vi "sendToAll.vi"(8 "error in (no error)":errorcluster, 9 "Data":u8[](array[numeric]), 10 "TCPok":bool[](array[boolean]), 11 "TCPconns":refnum<k5>[](array[refnum])) -> (0 "error out":errorcluster, 2 "activeTCP":bool[](array[boolean]))   [LabVIEW 2014]
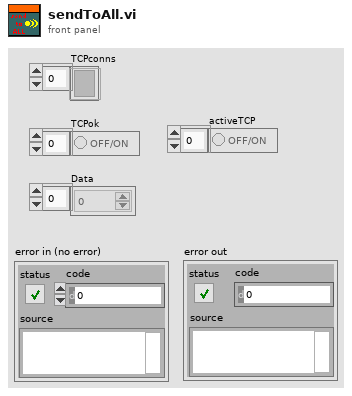
[diagram p1: front panel]
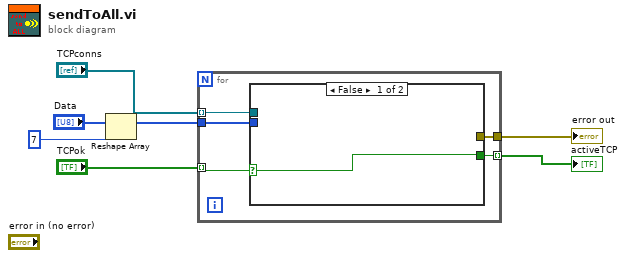
[diagram p0: block diagram]
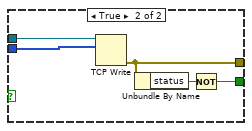
[diagram p2: hidden frame]
diagram:
  n1 = Reshape Array("Data", 7 ("dimension size")) -> (w2:u8[])
  n2 = for {
    tunnel: [w12] -> w3
    tunnel: "TCPconns" -> [w11] mode=indexing
    tunnel: "TCPok" -> [w10] mode=indexing
    tunnel: w2 -> [w9]
    tunnel: [w8] -> w7 mode=indexing
    n3 = case shown="False" w10 {
      selector: w10 -> [w13 _]
      tunnel: [_ w16] -> w12
      tunnel: w11 -> [_ w18]
      tunnel: w9 -> [_ w17]
      tunnel: [w13 w14] -> w8
      frame False {
      }
      frame True {
        n4 = TCP Write(connection ID=w18, data in=w17) -> (error out=w16:errorcluster)  [unwired: 2 in, 2 out]
        n5 = Unbundle By Name(w16) -> ("status"=w15:bool)
        n6 = Not(x=w15) -> (.not. x?=w14:bool)
      }
    }
  }
  "activeTCP" <- w7
  "error out" <- w3
